vi "Serial_log_build.vi"(1 "Read":string, 2 "Write String":string, 3 "Port Name":string) -> (0 "Output Array":string[](array[string]))   [LabVIEW 2010]
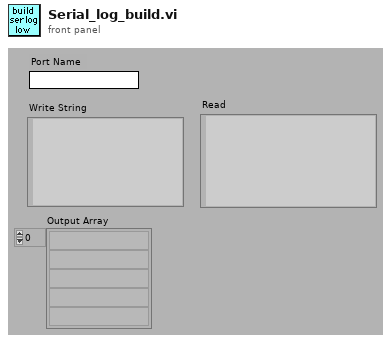
[diagram p1: front panel]
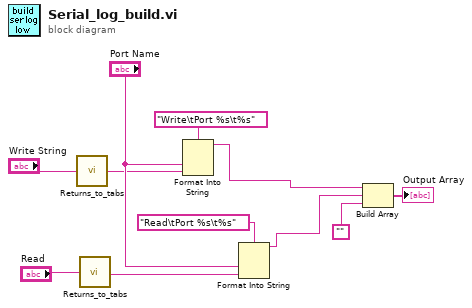
[diagram p0: block diagram]
diagram:
  n1 = call "Returns_to_tabs.vi"("Input string"="Write String") -> ("Output string"=w9:string)
  n2 = call "Returns_to_tabs.vi"("Input string"="Read") -> ("Output string"=w5:string)
  n3 = Format Into String(format string="Write\tPort %s\t%s" ("Format String"), "Port Name", w9) -> (resulting string=w7:string)  [unwired: 2 in, 1 out]
  n4 = Format Into String(format string="Read\tPort %s\t%s" ("Format String"), "Port Name", w5) -> (resulting string=w4:string)  [unwired: 2 in, 1 out]
  n5 = Build Array(w7, w4, "") -> (→"Output Array":string[])
